vi "MainCamera_simulation2.vi"() -> ()   [LabVIEW 2018]
uses:
  <vilib>/addons/lvgpu/lvcufft/CUFFT Type (cufftType).ctl
  <vilib>/Analysis/baseanly.llb/Real Outer Product.vi
  <vilib>/Analysis/Matrix/Numeric/Conversions/Matrix To Array - RM.vi
  <vilib>/addons/lvgpu/lvcufft/Create 2D FFT Plan.vi
  <vilib>/addons/lvgpu/lvcuda/CUDA CSG Device Ptr/Download 2D Data.vi
  <vilib>/addons/lvgpu/lvcufft/Complex FFT (CSG).vi
  <vilib>/addons/lvgpu/lvcuda/CUDA CSG Device Ptr/Upload 2D Data.vi
  <vilib>/addons/lvgpu/lvcuda.lvlib
  <vilib>/addons/lvgpu/lvcufft.lvlib
  <vilib>/Analysis/NI_AALBase.lvlib
  <vilib>/Analysis/Matrix/NI_Matrix.lvlib
  <vilib>/addons/lvgpu/lvcuda/CUDA CSG Device Ptr/CUDA CSG Device Ptr.lvclass
panel:
  out "Intensity Graph 2":sgl[][](graph)
  out "Intensity Graph":sgl[][](graph)
  out "error out":errorcluster
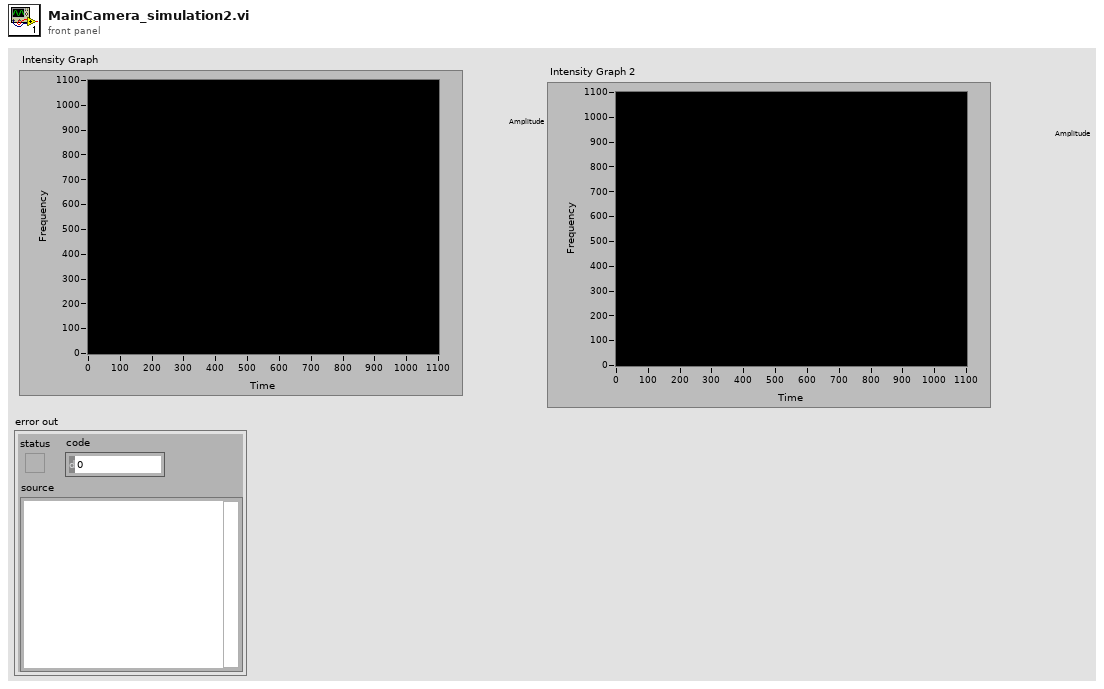
[diagram p1: front panel]
types:
  T1 = typedef "lvcufft.lvlib/CUFFT Type (cufftType).ctl" = i32
  T2 = typedef "NI_Matrix.lvlib/RealMatrix.ctl" = dbl[][]
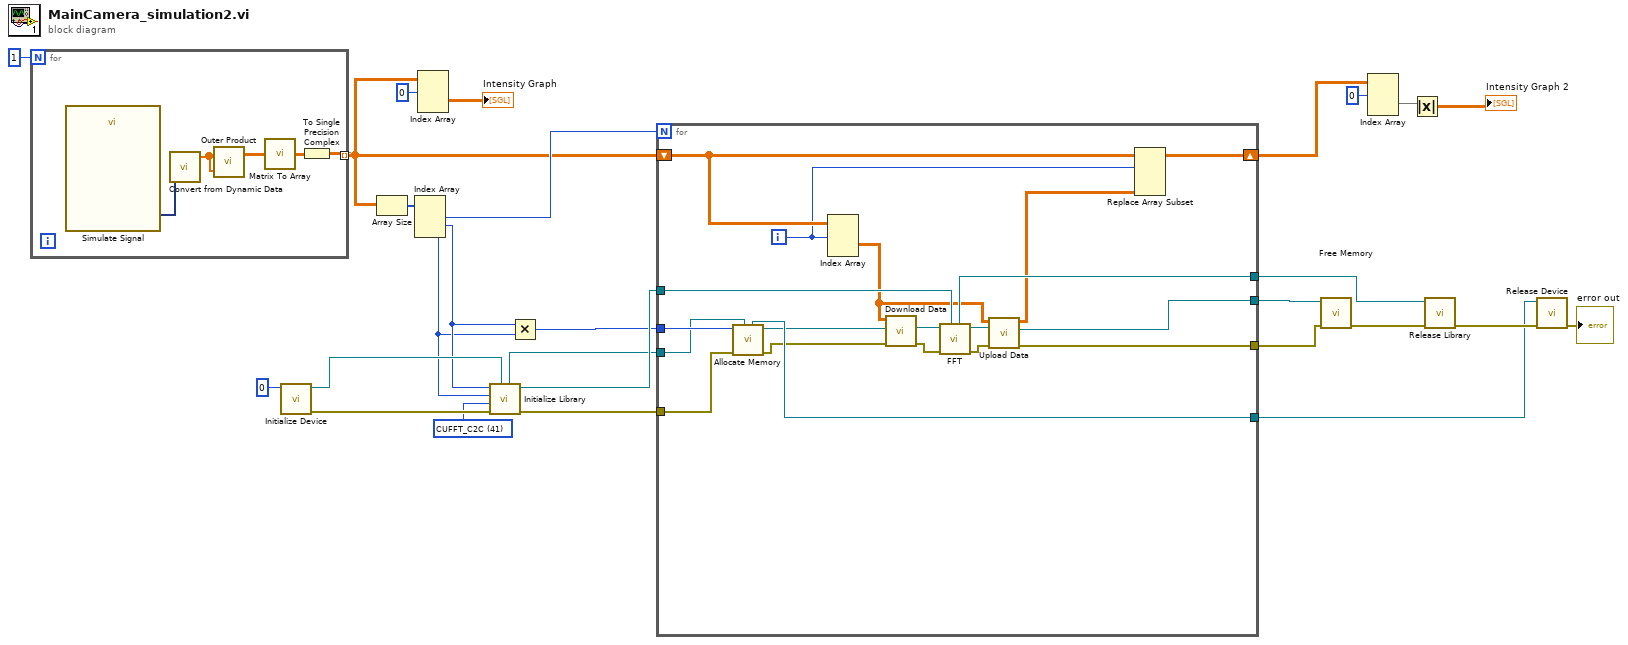
[diagram p0: block diagram]
diagram:
  w22 = T1 41 items=["CUFFT_R2C"=42, "CUFFT_C2R"=44, "CUFFT_C2C"=41, "CUFFT_D2Z"=106, "CUFFT_Z2D"=108, "CUFFT_Z2Z"=105] ("type")
  n1 = for {
    N: 1 -> [_]
    tunnel: [w28] -> w10 mode=indexing
    n2 = call "Simulate Signal"() -> ("Sine with Inverse F Noise"=w31:dynamicdata)  [unwired: 14 in, 1 out]
    n3 = call "Convert from Dynamic Data"("Dynamic Data Type"=w31) -> ("Array"=w32:dbl[])  [unwired: 3 in]
    n4 = call-poly <vilib>:"Outer Product.vi"("Y Vector"=w32, "X Vector"=w32) -> ("Outer Product"=w30:T2)  [unwired: 1 out]
    n5 = call-poly <vilib>:"Matrix To Array.vi"("Real Matrix"=w30) -> ("Real 2D Array"=w29:dbl[][])
    n6 = To Single Precision Complex(1:w29) -> (0:w28:csg[][])
  }
  n7 = call <vilib>:"Initialize Device.vi"("CUDA Device ID"=0) -> ("error out"=w24:errorcluster, "CUDA Context"=w25:refnum<class "CUDA Context.lvclass">)  [unwired: 8 in, 1 out]
  n8 = Array Size(array=w10) -> (size(s)=w20:i32[])
  n9 = Index Array(array=w20) -> (element #1=w19:i32, element #2=w18:i32, element #3=w17:i32)  [unwired: 3 in]
  n10 = Index Array(array=w10, index (dim 0)=0 ("index (page)")) -> (element=→"Intensity Graph":csg[][])  [unwired: 2 in]
  n11 = call-poly <vilib>:"Initialize Library.vi"("CUDA Context in"=w25, "error in"=w24, "type"=w22, "columns"=w17, "rows"=w18) -> ("error out"=w1:errorcluster, "CUFFT Handle"=w13:refnum<class "CUFFT Handle.lvclass">, "CUDA Context out"=w2:refnum<class "CUDA Context.lvclass">)  [unwired: 3 in, 1 out]
  n12 = Multiply(x=w18, y=w17) -> (x*y=w3:i32)
  n13 = for {
    N: w19 -> [_]
    tunnel: w3 -> [w51]
    tunnel: w2 -> [w50]
    shift-right: [w48] -> w7
    shift-left: w10 -> [w49]
    tunnel: [w47] -> w14
    tunnel: [w44] -> w16
    tunnel: [w42] -> w15
    tunnel: w13 -> [w41]
    tunnel: [w40] -> w12
    tunnel: w1 -> [w38]
    i -> [w43]
    n14 = call-poly <vilib>:"Allocate Memory.vi"("CUDA Context in"=w50, "error in"=w38, "size in elements"=w51) -> ("error out"=w46:errorcluster, "CUDA CSG Device Ptr out"=w37:refnum<class "CUDA CSG Device Ptr.lvclass">, "CUDA Context out"=w47:refnum<class "CUDA Context.lvclass">)  [unwired: 6 in]
    n15 = Index Array(array=w49, index (dim 0)=w43) -> (element=w34:csg[][])  [unwired: 2 in]
    n16 = call-poly <vilib>:"Download Data.vi"("error in"=w46, "dst in"=w37, "src in"=w34) -> ("error out"=w39:errorcluster, "dst out"=w35:refnum<class "CUDA CSG Device Ptr.lvclass">)  [unwired: 6 in, 1 out]
    n17 = call-poly <vilib>:"FFT.vi"("CUFFT Handle in"=w41, "error in"=w39, "signals in"=w35) -> ("error out"=w45:errorcluster, "spectrums out"=w36:refnum<class "CUDA CSG Device Ptr.lvclass">, "CUFFT Handle out"=w40:refnum<class "CUFFT Handle.lvclass">)  [unwired: 6 in]
    n18 = call-poly <vilib>:"Upload Data.vi"("error in"=w45, "src in"=w36, "dst in"=w34) -> ("error out"=w44:errorcluster, "src out"=w42:refnum<class "CUDA CSG Device Ptr.lvclass">, "dst out"=w33:csg[][])  [unwired: 6 in]
    n19 = Replace Array Subset(array=w49, new element=w33, index (dim 0)=w43) -> (w48:csg[][][])  [unwired: 2 in]
  }
  n20 = call-poly <vilib>:"Free Memory.vi"("error in"=w16, "CUDA CSG Device Ptr in"=w15) -> ("error out"=w26:errorcluster)  [unwired: 9 in]
  n21 = Index Array(array=w7, index (dim 0)=0 ("index (page)")) -> (element=w5:csg[][])  [unwired: 2 in]
  n22 = Absolute Value(x=w5) -> (abs(x)=→"Intensity Graph 2":sgl[][])
  n23 = call <vilib>:"Release Library.vi"("error in"=w26, "CUFFT Handle in"=w12) -> ("error out"=w27:errorcluster)  [unwired: 9 in]
  n24 = call <vilib>:"Release Device.vi"("error in"=w27, "CUDA Context in"=w14) -> ("error out"=→"error out":errorcluster)  [unwired: 9 in]
